vi "NXT Find max value.vi"(0 "array":sgl[](array[numeric])) -> (1 "Max Value":i16, 2 "Index":i32)   [LabVIEW 2012]
doc: "This VI find the maximum value of an array and returns it."
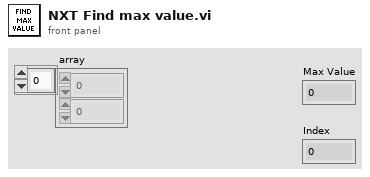
[diagram p1: front panel]
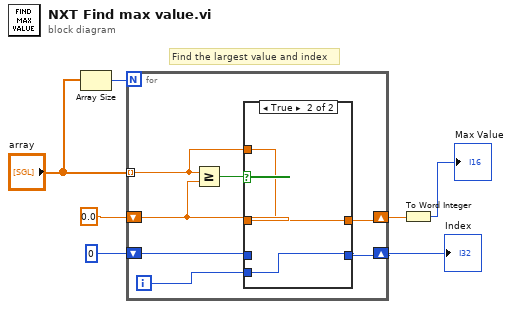
[diagram p0: block diagram]
diagram:
  # "Find the largest value and index"
  n1 = Array Size(array="array") -> (size(s)=w7:i32)
  n2 = for {
    N: w7 -> [_]
    tunnel: "array" -> [w8] mode=indexing
    shift-right: [w11] -> w2
    shift-left: sgl 0.0 -> [w13]
    shift-right: [w9] -> w3
    shift-left: 0 -> [w12]
    i -> [w10]
    n3 = Greater Or Equal?(x=w8, y=w13) -> (x >= y?=w14:bool)
    n4 = case shown="True" w14 {
      tunnel: w13 -> [w16 _]
      tunnel: w12 -> [w15 _]
      tunnel: w8 -> [_ w18]
      tunnel: [w16 w18] -> w11
      tunnel: w10 -> [_ w17]
      tunnel: [w15 w17] -> w9
      frame False {
      }
      frame True {
      }
    }
  }
  "Index" <- w3
  n5 = To Word Integer(number=w2) -> (16bit integer=→"Max Value":i16)
